vi "DualGateSTS.vi"() -> ()   [LabVIEW 2021]
panel:
  in  "Tabs":enum32{"Main", "Attributes"}(tab)
  in  "Safety Limit 2 (V)":dbl
  in  "Basename":string
  in  "Start Gate 2 (V)":dbl
  in  "End Gate 2 (V)":dbl
  in  "Increment Gate 2 (V)":dbl
  in  "Stop":bool
  out "Current Gate Voltage 2 (V)":dbl
  in  "Attributes":string[][](array[string])
  # "Dual Gate STS"
  # "Gate 2 Parameters"
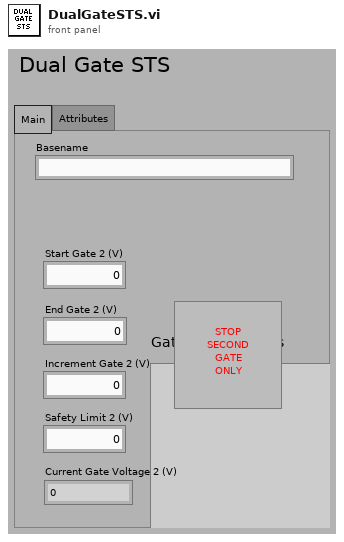
[diagram p1: front panel]
types:
  T1 = enum16{"Output 2 (V)", "Output 3 (V)", "Output 4 (V)"}
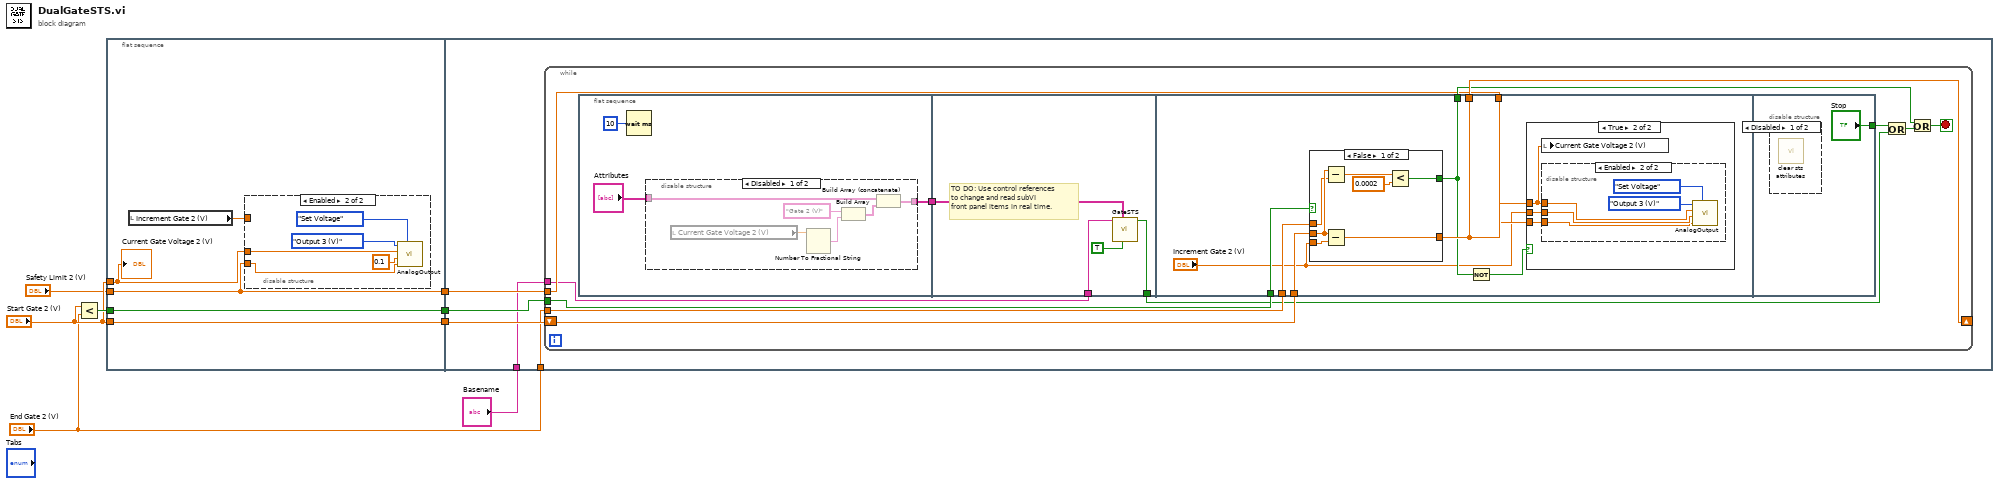
[diagram p0: block diagram]
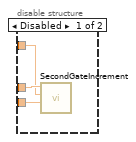
[diagram p2: hidden frame]
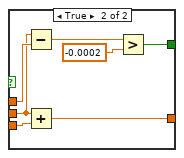
[diagram p4: hidden frame]
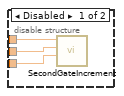
[diagram p6: hidden frame]
diagram:
  n1 = Less?(x="Start Gate 2 (V)", y="End Gate 2 (V)") -> (x < y?=w8:bool)
  n2 = flat-sequence {
    tunnel: [w13] -> w4
    tunnel: [w12] -> w3
    tunnel: [w11] -> w2
    tunnel: "Safety Limit 2 (V)" -> [w11]
    tunnel: "Start Gate 2 (V)" -> [w10]
    tunnel: "Start Gate 2 (V)" -> [w12]
    tunnel: w8 -> [w13]
    tunnel: w4 -> [w26]
    tunnel: w3 -> [w25]
    tunnel: "End Gate 2 (V)" -> [w24]
    tunnel: w2 -> [w23]
    tunnel: "Basename" -> [w22]
    frame #0 {
      n3 = local read "Increment Gate 2 (V)"() -> (w9:dbl)
      n4 = disable-structure shown="Enabled" {
        disable-tunnel: w11 -> [w16 w20]
        disable-tunnel: w10 -> [w15 w21]
        disable-tunnel: w9 -> [w14 _]
        frame Disabled {
          n5 = call "SecondGateIncrement.vi"("Voltage Safety Limit"=w16, "Increment"=w14, "Gate Voltage"=w15) -> ()  [unwired: 9 in]
        }
        frame Enabled {
          n6 = call "AnalogOutput.vi"("Read or Set Voltage?"=enum16{"Read Voltage", "Set Voltage"}."Set Voltage", "Voltage Safety Limit"=w20, "Increment"=0.1, "Target Voltage"=w21, "Channel"=T1."Output 3 (V)") -> ()  [unwired: 6 in, 1 out]
        }
      }
      "Current Gate Voltage 2 (V)" <- w10
    }
    frame #1 {
      n7 = while {
        tunnel: w26 -> [w33]
        shift-right: [w37] -> _
        shift-left: w25 -> [w35]
        tunnel: w24 -> [w34]
        tunnel: w23 -> [w32]
        tunnel: w22 -> [w31]
        stop <- w38 stop-if-true
        n8 = flat-sequence {
          tunnel: [w39] -> w30
          tunnel: w31 -> [w51]
          tunnel: w30 -> [w52]
          tunnel: [w50] -> w29
          tunnel: [w60] -> w37
          tunnel: [w59] -> w36
          tunnel: w35 -> [w58]
          tunnel: w34 -> [w57]
          tunnel: w33 -> [w56]
          tunnel: w32 -> [w54]
          tunnel: ["Stop"] -> w27
          frame #0 {
            n9 = Wait (ms)(milliseconds to wait=u32 10) -> ()  [unwired: 1 out]
            n10 = disable-structure shown="Disabled" {
              disable-tunnel: "Attributes" -> [w45 w48]
              disable-tunnel: [w42 w48] -> w39
              frame Disabled {
                n11 = local read "Current Gate Voltage 2 (V)"() -> (w46:dbl)
                n12 = Number To Fractional String(number=w46) -> (F-format string=w47:string)  [unwired: 3 in]
                n13 = Build Array("Gate 2 (V)" ("element"), w47) -> (w44:string[])
                n14 = Build Array (concatenate)(w45, w44) -> (w42:string[][])
              }
              frame Enabled {
              }
            }
          }
          frame #1 {
            # "TO DO: Use control references\nto change and read subVI\nfront panel items in real time."
            n15 = call "GateSTS.vi"("Store\nSecond Gate?"=TRUE ("Store\nSecond Gate?"), "Attributes"=w52, "Basename"=w51) -> ("Stop Loop"=w50:bool)  [unwired: 7 in]
          }
          frame #2 {
            n16 = case shown="False" w56 {
              tunnel: w58 -> [w65 w71]
              tunnel: "Increment Gate 2 (V)" -> [w66 w74]
              tunnel: [w67 w73] -> w60
              tunnel: w57 -> [w64 w72]
              tunnel: [w62 w70] -> w59
              frame False {
                n17 = Subtract(x=w65, y=w64) -> (x-y=w63:dbl)
                n18 = Subtract(x=w65, y=w66) -> (x-y=w67:dbl)
                n19 = Less?(x=w63, y=0.0002) -> (x < y?=w62:bool)
              }
              frame True {
                n20 = Subtract(x=w71, y=w72) -> (x-y=w69:dbl)
                n21 = Add(x=w71, y=w74) -> (x+y=w73:dbl)
                n22 = Greater?(x=w69, y=-0.0002) -> (0:w70:bool)
              }
            }
            n23 = Not(x=w59) -> (.not. x?=w55:bool)
            n24 = case shown="True" w55 {
              tunnel: w60 -> [_ w77]
              tunnel: w54 -> [_ w76]
              tunnel: "Increment Gate 2 (V)" -> [_ w75]
              frame False {
              }
              frame True {
                n25 = local write "Current Gate Voltage 2 (V)"(w77) -> ()
                n26 = disable-structure shown="Enabled" {
                  disable-tunnel: w77 -> [w80 w85]
                  disable-tunnel: w76 -> [w79 w83]
                  disable-tunnel: w75 -> [w78 w84]
                  frame Disabled {
                    n27 = call "SecondGateIncrement.vi"("Voltage Safety Limit"=w79, "Increment"=w78, "Gate Voltage"=w80) -> ()  [unwired: 9 in]
                  }
                  frame Enabled {
                    n28 = call "AnalogOutput.vi"("Read or Set Voltage?"=enum16{"Read Voltage", "Set Voltage"}."Set Voltage", "Voltage Safety Limit"=w83, "Increment"=w84, "Target Voltage"=w85, "Channel"=T1."Output 3 (V)") -> ()  [unwired: 6 in, 1 out]
                  }
                }
              }
            }
          }
          frame #3 {
            n29 = disable-structure shown="Disabled" {
              frame Disabled {
                n30 = call "clear sts attributes.vi"() -> ()  [unwired: 12 in]
              }
              frame Enabled {
              }
            }
          }
        }
        n31 = Or(x=w27, y=w29) -> (x .or. y?=w28:bool)
        n32 = Or(x=w36, y=w28) -> (x .or. y?=w38:bool)
      }
    }
  }
